vi "sinefunction.vi"(3 "output control":T1, 4 "data":variant, 5 "X":dbl[](array[numeric]), 6 "Coefficients":dbl[](array[numeric])) -> (0 "error out":errorcluster, 1 "f'(X,a)":dbl[][](array[numeric]), 2 "f(X,a)":dbl[](array[numeric]))   [LabVIEW 2014]
uses:
  <vilib>/gmath/NumericalOptimization/LM_output select.ctl
  <vilib>/gmath/NI_Gmath.lvlib
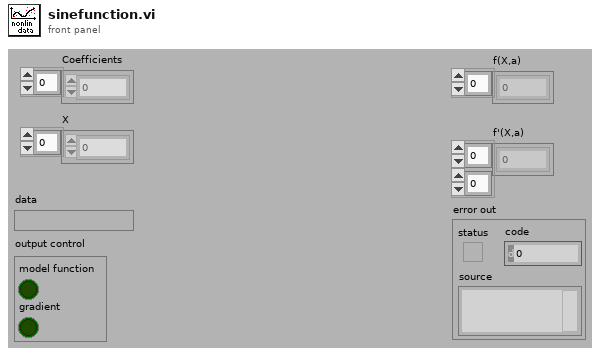
[diagram p1: front panel]
types:
  T1 = typedef "NI_Gmath.lvlib/LM_output select.ctl" = cluster{"model function":bool, "gradient":bool}
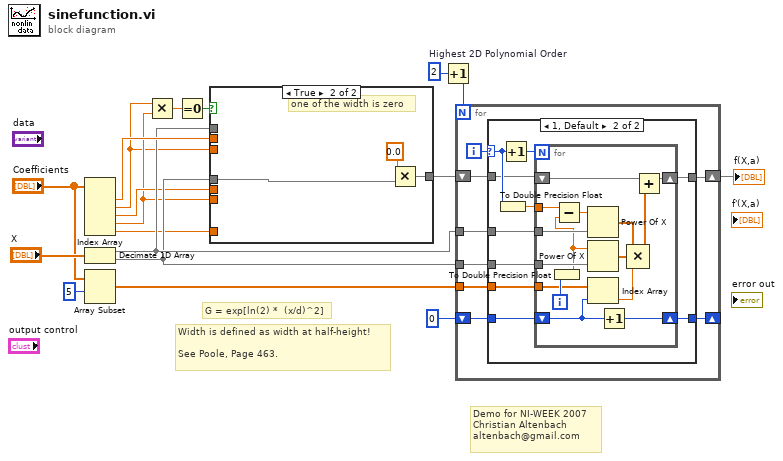
[diagram p0: block diagram]
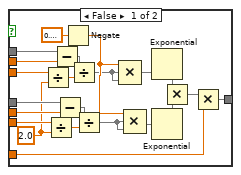
[diagram p2: hidden frame]
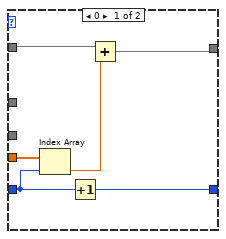
[diagram p3: hidden frame]
diagram:
  w2 = 2  # Highest 2D Polynomial Order
  # "Demo for NI-WEEK 2007\nChristian Altenbach\naltenbach@gmail.com"
  # "G = exp[ln(2) *  (x/d)^2]"
  # "Width is defined as width at half-height!\n\nSee Poole, Page 463."
  n1 = Index Array(array="Coefficients") -> (element #1=w17:dbl, element #2=w5:dbl, element #3=w14:dbl, element #4=w13:dbl, element #5=w4:dbl)  [unwired: 5 in]
  n2 = Decimate 1D Array("X") -> (w16:dbl[], w15:dbl[])
  n3 = Array Subset(array="Coefficients", index=5) -> (w8:dbl[])  [unwired: 1 in]
  n4 = Multiply(x=w5, y=w13) -> (x*y=w12:dbl)
  n5 = Equal To 0?(x=w12) -> (x = 0?=w11:bool)
  n6 = case shown="True" w11 {
    tunnel: w17 -> [w40 _]
    tunnel: w16 -> [w39 _]
    tunnel: w5 -> [w38 _]
    tunnel: w15 -> [w37 w41]
    tunnel: w14 -> [w36 _]
    tunnel: w13 -> [w33 _]
    tunnel: [w30 w42] -> w10
    tunnel: w4 -> [w29 _]
    frame False {
      w31 = 2.0 ("y")
      n7 = Divide(x=w38, y=w31) -> (x/y=w34:dbl)
      n8 = Divide(x=w33, y=w31) -> (x/y=w32:dbl)
      n9 = Subtract(x=w39, y=w40) -> (x-y=w24:dbl[])
      n10 = Subtract(x=w37, y=w36) -> (x-y=w23:dbl[])
      n11 = Negate(x=0.6931471805599453) -> (-x=w27:dbl)
      n12 = Divide(x=w24, y=w34) -> (x/y=w25:dbl[])
      n13 = Divide(x=w23, y=w32) -> (x/y=w22:dbl[])
      n14 = Compound Arithmetic op=MULTIPLY(w27, w25, w25) -> (w26:dbl[])
      n15 = Compound Arithmetic op=MULTIPLY(w27, w22, w22) -> (w21:dbl[])
      n16 = Exponential(1:w26) -> (0:w19:dbl[])
      n17 = Exponential(1:w21) -> (0:w20:dbl[])
      n18 = Multiply(x=w19, y=w20) -> (x*y=w35:dbl[])
      n19 = Multiply(x=w35, y=w29) -> (x*y=w30:dbl[])
    }
    frame True {
      # "one of the width is zero"
      n20 = Multiply(x=0.0, y=w41) -> (x*y=w42:dbl[])
    }
  }
  n21 = Increment(x=w2) -> (x+1=w1:i32)
  n22 = for {
    N: w1 -> [_]
    tunnel: w16 -> [w49]
    tunnel: w15 -> [w51]
    tunnel: w8 -> [w48]
    shift-right: [w46] -> _
    shift-left: 0 -> [w47]
    shift-right: [w44] -> w6
    shift-left: w10 -> [w45]
    i -> [w50]
    n23 = case shown="1, Default" w50 {
      selector: w50 -> [_ w64]
      tunnel: w51 -> [_ w67]
      tunnel: w49 -> [_ w66]
      tunnel: w48 -> [w57 w63]
      tunnel: w47 -> [w56 w62]
      tunnel: [w55 w61] -> w46
      tunnel: w45 -> [w53 w60]
      tunnel: [w54 w59] -> w44
      frame 0 {
        n24 = Index Array(array=w57, index=w56) -> (element=w52:dbl)
        n25 = Increment(x=w56) -> (x+1=w55:i32)
        n26 = Add(x=w53, y=w52) -> (x+y=w54:dbl[])
      }
      frame 1, Default {
        n27 = To Double Precision Float(number=w64) -> (double precision float=w58:dbl)
        n28 = Increment(x=w64) -> (x+1=w65:i32)
        n29 = for {
          N: w65 -> [_]
          tunnel: w67 -> [w82]
          tunnel: w66 -> [w81]
          tunnel: w58 -> [w80]
          tunnel: w63 -> [w75]
          shift-right: [w73] -> w61
          shift-left: w62 -> [w74]
          shift-right: [w70] -> w59
          shift-left: w60 -> [w71]
          i -> [w76]
          n30 = To Double Precision Float(number=w76) -> (double precision float=w68:dbl)
          n31 = Subtract(x=w80, y=w68) -> (x-y=w77:dbl)
          n32 = Power Of X(1:w81, 2:w77) -> (0:w79:dbl[])
          n33 = Power Of X(1:w82, 2:w68) -> (0:w78:dbl[])
          n34 = Index Array(array=w75, index=w74) -> (element=w72:dbl)
          n35 = Increment(x=w74) -> (x+1=w73:i32)
          n36 = Compound Arithmetic op=MULTIPLY(w79, w78, w72) -> (w69:dbl[])
          n37 = Add(x=w71, y=w69) -> (x+y=w70:dbl[])
        }
      }
    }
  }
  "f(X,a)" <- w6
